vi "PH_AxisGUI_BaseClass.DisableAxisControl.vi"(0 "i ref in":refnum<vi>, 1 "Axis":i32, 2 "Disabled":T1(ring), 5 "error in":errorcluster) -> (14 "i ref out":refnum<vi>, 19 "error out":errorcluster)   [LabVIEW 2014, in "PH_AxisGUI_BaseClass.lvlib"]
doc: "THIS VI acts on GUI Elements."
uses:
  PH_AxisGUI_BaseClass.lvlib
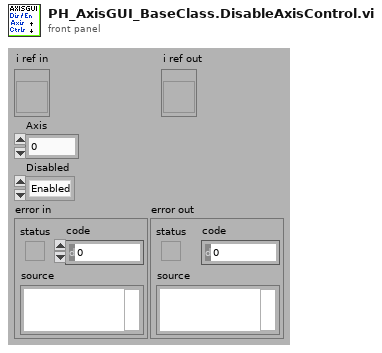
[diagram p1: front panel]
types:
  T1 = enum8{"Enabled", "Disabled", "Disabled and Grayed Out"}
  T2 = typedef "PH_AxisGUI_BaseClass.lvlib/PH_AxisGUI_BaseClass.i attribute.ctl" = cluster{"Axes":T3[]}
  T3 = typedef "PH_AxisGUI_BaseClass.lvlib/PH_AxisGUI_BaseClass.Axis Attributes.ctl" = cluster{"Axis GUI Refs":T4, "Address":T5, "Name":string, "Label \"Back\"":string, "Labell \"Forth\"":string, "Moving?":bool}
  T4 = typedef "PH_AxisGUI_BaseClass.lvlib/PH_AxisGUI_BaseClass.Axis GUI Refs.ctl" = cluster{"Back":refnum<vi>, "Forth":refnum<vi>, "Status":refnum<vi>, "Target":refnum<vi>, "Address":refnum<vi>, "Status Bar":refnum<vi>, "Settings":refnum<vi>, "Activity":refnum<vi>, "Clear Error":refnum<vi>}
  T5 = typedef "PH_Stepmotor_BaseClass.lvlib/PH_Stepmotor_BaseClass.Axis Address.ctl" = cluster{"Instance":string, "Motor Nr":i32}
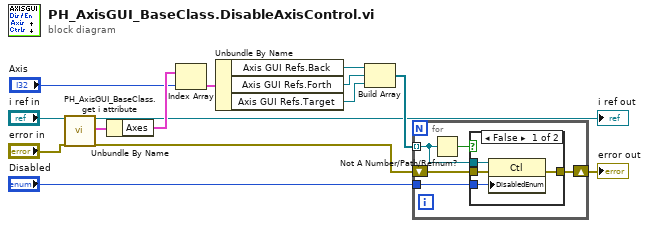
[diagram p0: block diagram]
diagram:
  n1 = call "PH_AxisGUI_BaseClass.get i attribute.vi"("i ref in"="i ref in", "error in (no error)"="error in") -> ("i ref out"=→"i ref out":refnum<vi>, "i attribute"=w9:T2, "error out"=w10:errorcluster)  [unwired: 15 in]
  n2 = Unbundle By Name(w9) -> ("Axes"=w8:T3[])
  n3 = Index Array(array=w8, index="Axis") -> (element=w4:T3)
  n4 = Unbundle By Name(w4) -> ("Axis GUI Refs.Back"=w3:refnum<vi>, "Axis GUI Refs.Forth"=w2:refnum<vi>, "Axis GUI Refs.Target"=w1:refnum<vi>)
  n5 = Build Array(w3, w2, w1) -> (w11:refnum<vi>[])
  n6 = for {
    shift-right: [w18] -> w13
    shift-left: w10 -> [w19]
    tunnel: w11 -> [w15] mode=indexing
    tunnel: "Disabled" -> [w17]
    n7 = Not A Number/Path/Refnum?(number/path/refnum=w15) -> (NaN/Path/Refnum?=w16:bool)
    n8 = case shown="False" w16 {
      tunnel: w19 -> [w23 w24]
      tunnel: [w22 w24] -> w18
      tunnel: w15 -> [w21 _]
      tunnel: w17 -> [w20 _]
      frame False {
        n9 = property class="Ctl"(reference=w21, error in=w23, "DisabledEnum"=w20) -> (error out=w22:errorcluster)  [unwired: 1 out]
      }
      frame True {
      }
    }
  }
  "error out" <- w13
